vi "rec_jumperDAQreplicates_v03.vi"(0 "AI task in":refnum<k21>, 1 "which clamp":enum16{"VClamp", "IClamp"}(ring), 5 "number of samples":i32=-1, 7 "Duration (s)":dbl, 9 "AO task in":refnum<k21>, 11 "error in":errorcluster) -> (4 "AI task out":refnum<k21>, 6 "data out (pA or mV)":waveform(dbl)(graph), 10 "AO task out":refnum<k21>, 15 "error out":errorcluster)   [LabVIEW 2019]
uses:
  <vilib>/DAQmx/read.llb/DAQmx Read (Analog Wfm 1Chan NSamp).vi
  <vilib>/DAQmx/miscellaneous.llb/DAQmx Fill In Error Info.vi
  <resource>/objmgr/daqmx.rc
panel:
  out "AvailSampPerChan":u32
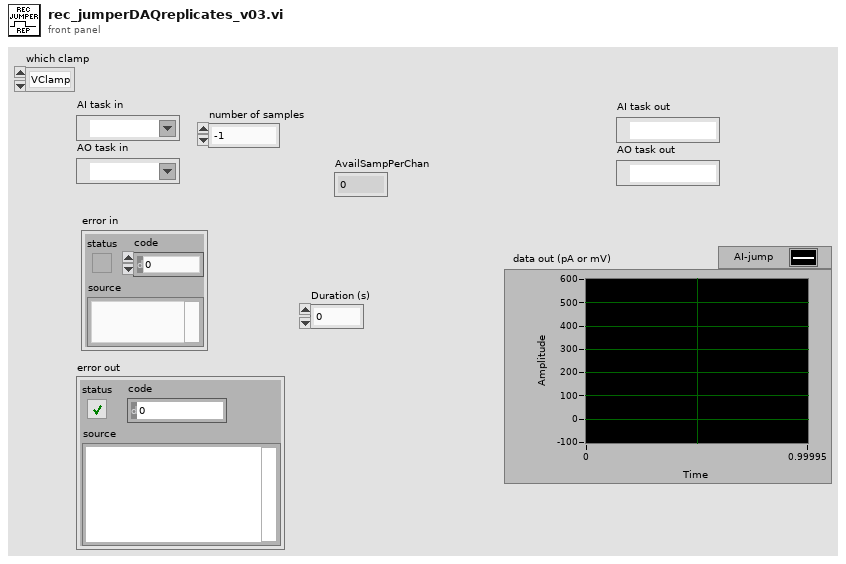
[diagram p1: front panel]
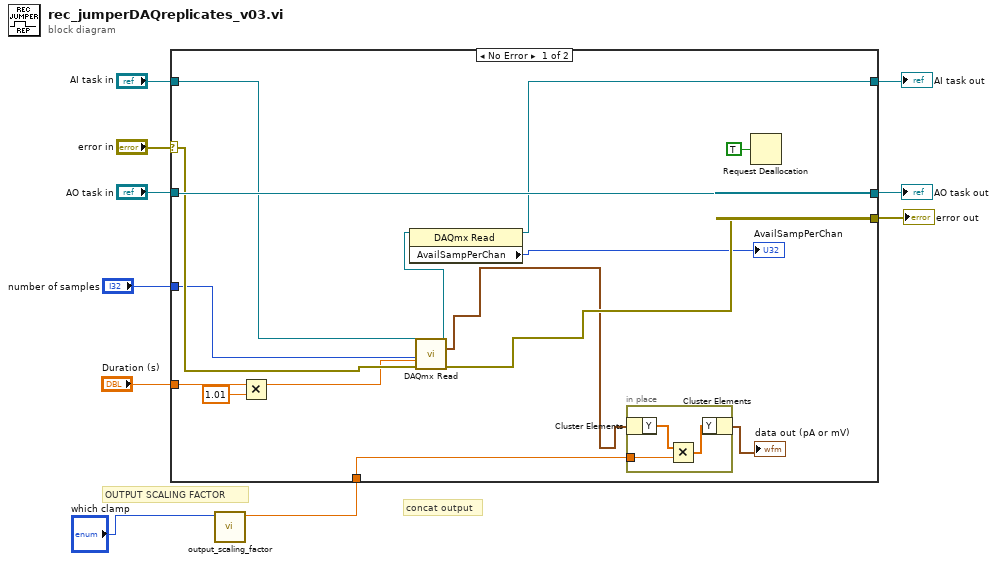
[diagram p0: block diagram]
diagram:
  # "concat output"
  # "OUTPUT SCALING FACTOR"
  n1 = call "output_scaling_factor.vi"("which clamp"="which clamp") -> ("output scaling factor"=w5:dbl)  [unwired: 10 in]
  n2 = case shown="No Error" "error in" {
    selector: "error in" -> [w22 w30]
    tunnel: "AI task in" -> [w23 w29]
    tunnel: "AO task in" -> [w25 w31]
    tunnel: [w25 w31] -> w7
    tunnel: [w18 w29] -> w3
    tunnel: [w20 w30] -> w6
    tunnel: w5 -> [w24 _]
    tunnel: "number of samples" -> [w21 _]
    tunnel: "Duration (s)" -> [w17 _]
    frame No Error {
      n3 = Multiply(x=w17, y=1.01) -> (x*y=w16:dbl)
      n4 = call-poly <vilib>:"DAQmx Read.vi"("task/channels in"=w23, "number of samples per channel"=w21, "timeout"=w16, "error in"=w22) -> ("task out"=w13:refnum<k21>, "data"=w12:waveform(dbl), "error out"=w20:errorcluster)  [unwired: 9 in]
      n5 = property class="DAQmx Read"(reference=w13) -> (reference out=w18:refnum<k21>, "AvailSampPerChan"=→"AvailSampPerChan":u32)  [unwired: 1 in, 1 out]
      n6 = in-place {
        in-place-border: w24 -> [w28]
        n7 = in-place-cluster #1(w12) -> ("Y"=w27:dbl[])
        n8 = Multiply(x=w27, y=w28) -> (x*y=w26:dbl[])
        n9 = in-place-cluster #1("Y"=w26) -> (→"data out (pA or mV)":waveform(dbl))
      }
      n10 = Request Deallocation(TRUE ("flag")) -> ()
    }
    frame Error {
    }
  }
  "AI task out" <- w3
  "AO task out" <- w7
  "error out" <- w6
